vi "Trap1-02-06-2017.vi"() -> (4 "U":fxp<+/-,26,5> format="%.23g")   [LabVIEW 2010]
uses:
  <vilib>/eio/EIONode/EIONode.xnode
  <vilib>/rvi/eio/nirviEIOImplementation/nirviEIOImplementation.xnode
  <vilib>/rvi/eio/common/nirviEmuClasses.ctl
  <vilib>/rvi/FXPMathLib/FxpAdd/XNode/nifxpmath_Add.xnode
  <vilib>/rvi/FXPMathLib/FxpAdd/subVIs/nifxpmath_Add_SimConfig.ctl
  <vilib>/fxp/LVFixedPointQuantizationPolicyTypeDef.ctl
  <vilib>/fxp/LVFixedPointOverflowPolicyTypeDef.ctl
  <vilib>/rvi/FXPMathLib/FxpDiv/XNode/nifxpmath_Div.xnode
  <vilib>/rvi/FXPMathLib/FxpDiv/subVIs/nifxpmath_Div_SimConfig.ctl
  <vilib>/rvi/eio/common/nirviEmuTemplateMethod_noerrors.vi
  <vilib>/rvi/FXPMathLib/FxpAdd/simVIs/DllFxpAddTemp_sub.vi
  <vilib>/rvi/FXPMathLib/FxpDiv/simVIs/DllFxpDivTemp_sub.vi
panel:
  in  "t3(ms)":u32
  in  "t2(ms)":u32
  in  "heizen":bool
  in  "t1(ms)":u16
  in  "t0(ms)":u16
  in  "stop":bool
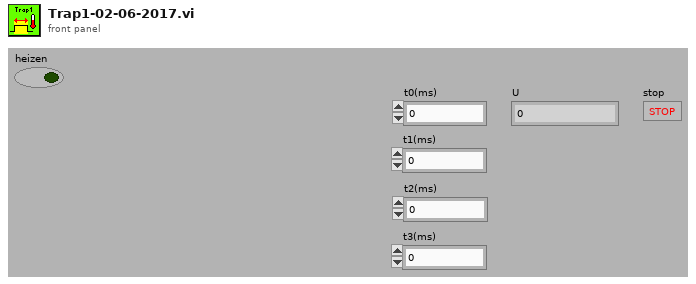
[diagram p1: front panel]
types:
  T1 = typedef "nirviEmuClasses.ctl" = enum16{"IO Read", "IO Write", "Method", "Property Read", "Property Write"}
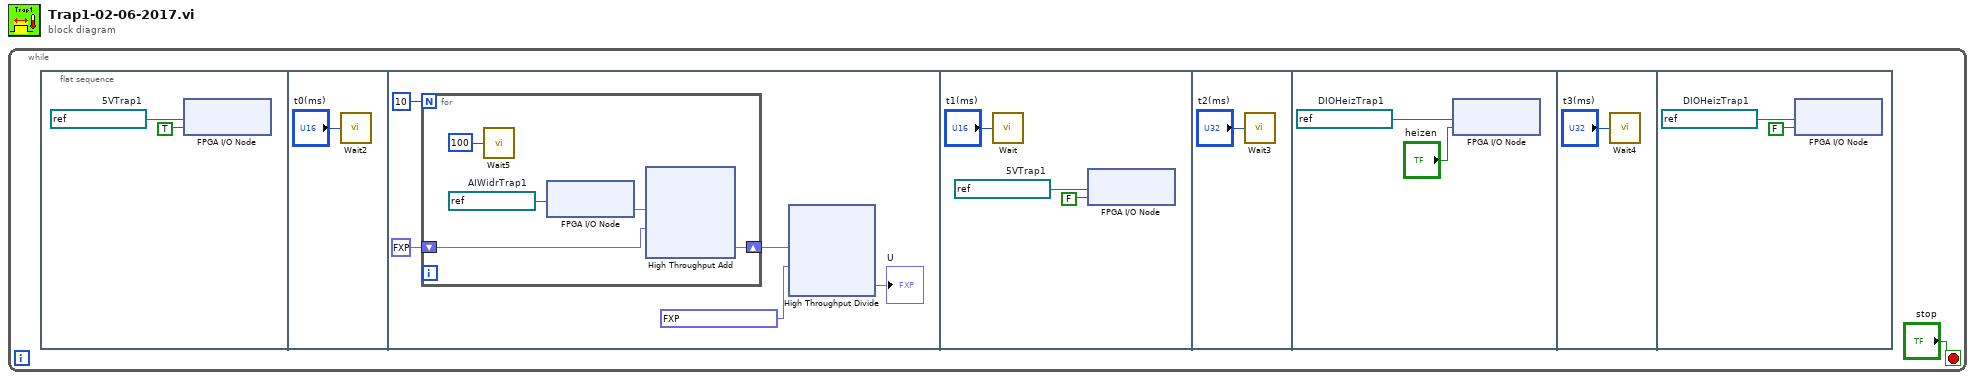
[diagram p0: block diagram]
diagram:
  n1 = while {
    stop <- "stop" stop-if-true
    n2 = flat-sequence {
      frame #0 {
        w3 = refnum<k21> "Mod6/DIO21"  # 5VTrap1
        n3 = xnode "FPGA I/O Node"("I/O Item"=TRUE, "FPGA I/O In"=w3) -> ()  [unwired: 1 out]
      }
      frame #1 {
        n4 = call "Wait2"("Count(uSec)"="t0(ms)") -> ()  [unwired: 1 out]
      }
      frame #2 {
        n5 = for {
          N: 10 -> [_]
          shift-right: [w48] -> w19
          shift-left: fxp<+/-,30,9> 0.0 ("x+y") -> [w49]
          w52 = refnum<k21> "Mod1/AI30"  # AIWidrTrap1
          n6 = call "Wait5"("Count(uSec)"=u8 100) -> ()  [unwired: 1 out]
          n7 = xnode "FPGA I/O Node"("FPGA I/O In"=w52) -> ("I/O Item"=w50:fxp<+/-,26,5>)  [unwired: 1 out]
          n8 = xnode "High Throughput Add"("x"=w50, "y"=w49) -> ("x+y"=w48:fxp<+/-,30,9>)
        }
        n9 = xnode "High Throughput Divide"("x"=w19, "y"=fxp<+/-,5,5> 10.0) -> ("x/y"=→"U":fxp<+/-,26,5>)
      }
      frame #3 {
        w103 = refnum<k21> "Mod6/DIO21"  # 5VTrap1
        n10 = call "Wait"("Count(uSec)"="t1(ms)") -> ()  [unwired: 1 out]
        n11 = xnode "FPGA I/O Node"("I/O Item"=FALSE, "FPGA I/O In"=w103) -> ()  [unwired: 1 out]
      }
      frame #4 {
        n12 = call "Wait3"("Count(uSec)"="t2(ms)") -> ()  [unwired: 1 out]
      }
      frame #5 {
        w118 = refnum<k21> "Mod6/DIO19"  # DIOHeizTrap1
        n13 = xnode "FPGA I/O Node"("I/O Item"="heizen", "FPGA I/O In"=w118) -> ()  [unwired: 1 out]
      }
      frame #6 {
        n14 = call "Wait4"("Count(uSec)"="t3(ms)") -> ()  [unwired: 1 out]
      }
      frame #7 {
        w132 = refnum<k21> "Mod6/DIO19"  # DIOHeizTrap1
        n15 = xnode "FPGA I/O Node"("I/O Item"=FALSE, "FPGA I/O In"=w132) -> ()  [unwired: 1 out]
      }
    }
  }
